vi "setBarFrameStyle.vi"(8 "Error In":errorcluster, 10 "style":T1 items=["NoFrame", "Plain", "Raised"], 11 "LQwtPlotBarChart In":refnum<class "LQwtPlotBarChart.lvclass">) -> (0 "Error Out":errorcluster, 3 "LQwtPlotBarChart Out":refnum<class "LQwtPlotBarChart.lvclass">)   [LabVIEW 2014, in "LQwtPlotBarChart.lvclass"]
doc: "LabVIEW-specific documentation is not yet available."
uses:
  LQwtPlotBarChart.lvclass
  Qwt/QwtColumnSymbol/FrameStyle.ctl
  LQ Core/LQIdentity/LQIdentity.lvclass/LQIdentity.ctl
  LQ Core/LQ Core.lvlib
  LQ Core/LQIdentity/LQIdentity.lvclass
  Qwt/QwtColumnSymbol/QwtColumnSymbol.lvclass
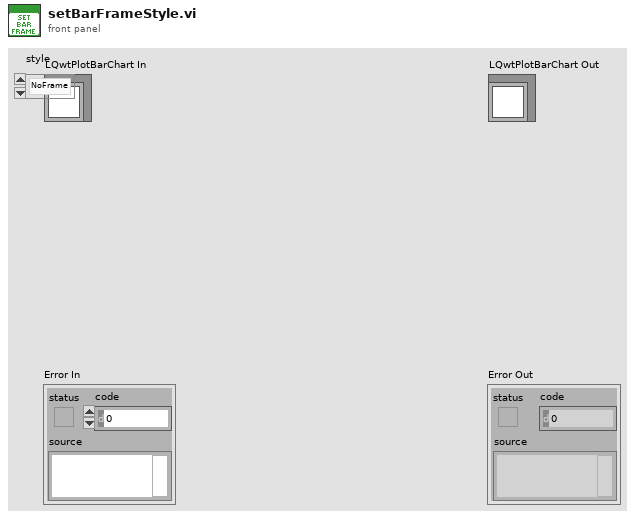
[diagram p1: front panel]
types:
  T1 = typedef "QwtColumnSymbol.lvclass/FrameStyle.ctl" = i32
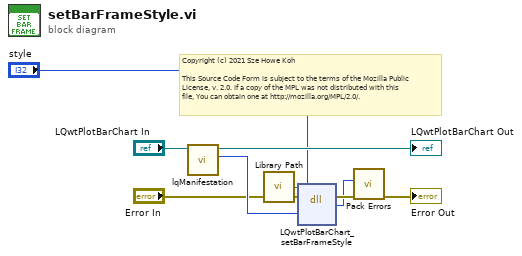
[diagram p0: block diagram]
diagram:
  # "Copyright (c) 2021 Sze Howe Koh\n\nThis Source Code Form is subject to the terms of the Mozilla Public\nLicense, v. 2.0. If a copy of the MPL was not distributed with this\nfile, You can obtain one at http://mozilla.org/MPL/2.0/."
  n1 = call "lqManifestation.vi"("LQIdentity in"="LQwtPlotBarChart In") -> ("Manifestation"=w6:u64, "LQIdentity out"=→"LQwtPlotBarChart Out":refnum<class "LQwtPlotBarChart.lvclass">)  [unwired: 9 in]
  n2 = call "Library Path.vi"() -> ("Library Path"=w7:path)
  n3 = dll-call lib="?" fn="LQwtPlotBarChart_setBarFrameStyle"(path in=w7, error in="Error In", "_instance"=w6, "style"="style") -> (error out=w4:errorcluster, w2:i32)  [unwired: 3 in, 1 out]
  n4 = call "Pack Errors.vi"("Error In"=w4, "Error Code"=w2) -> ("Error Out"=→"Error Out":errorcluster)  [unwired: 9 in]
